vi "SetOrigDly.vi"(8 "错误输入（无错误）":errorcluster, 10 "OrigDly":u32) -> (0 "错误输出":errorcluster)   [LabVIEW 2018]
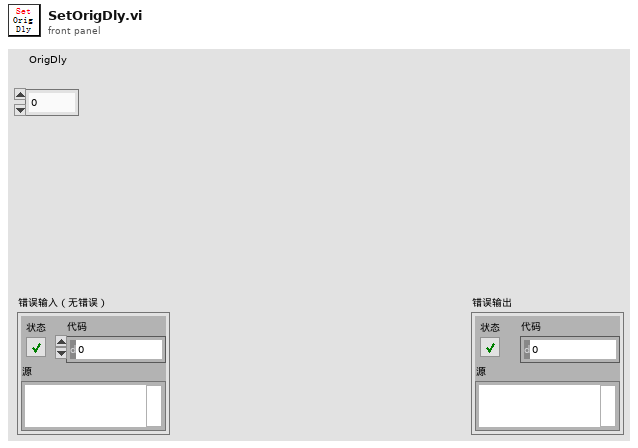
[diagram p1: front panel]
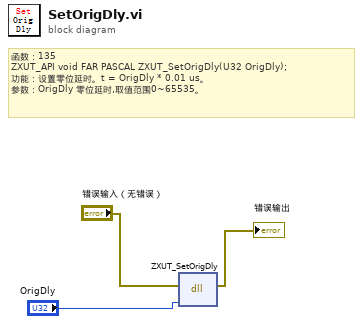
[diagram p0: block diagram]
diagram:
  # "函数：135\nZXUT_API void\tFAR PASCAL ZXUT_SetOrigDly(U32 OrigDly);\n功能：设置零位延时。t = OrigDly * 0.01 us。\n参数：OrigDly 零位延时,取值范围0~65535。"
  n1 = dll-call lib="PTH2Rabs E软件项目超声超声子VI函数VI\tTCG处理ZXUTConfigMgr.dll" fn="ZXUT_SetOrigDly"(error in="错误输入（无错误）", "OrigDly"="OrigDly") -> (error out=→"错误输出":errorcluster)  [unwired: 4 in, 1 out]
